vi "RGseriesSerial.vi"() -> ()   [LabVIEW 2009]
uses:
  <vilib>/Instr/_visa.llb/VISA Configure Serial Port (Instr).vi
panel:
  out "ICN MES COM":string
  out "VCN MES COM":string
  in  "On/Off":bool
  out "VCN MES":string
  in  "VISA resource name":refnum<visa-resource-name>
  in  "timeout (10sec)":u32=10000
  out "ICN MES":string
  out "VCN_REQ_COM":string
  out "ICN_REQ_COM":string
  in  "VCN_REQ":dbl
  in  "ICN_REQ":dbl(knob) scale=0.0..3.0
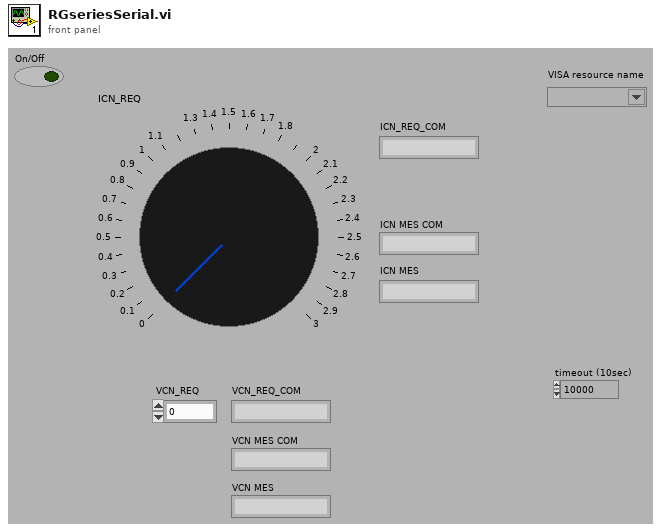
[diagram p1: front panel]
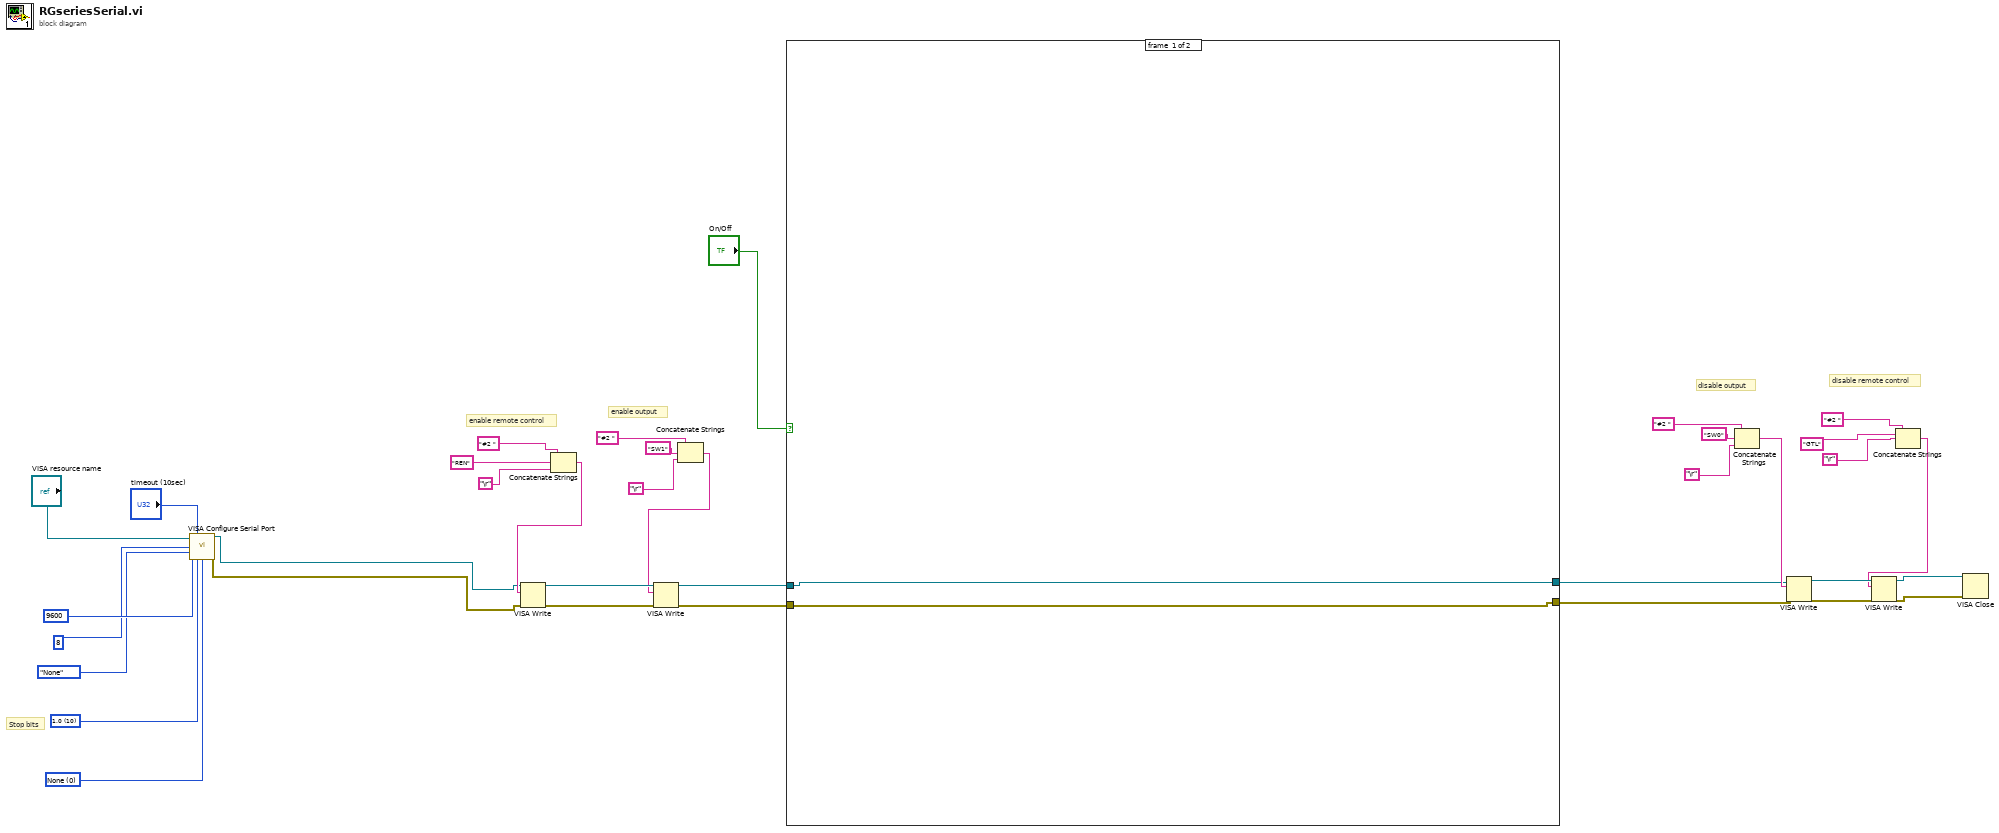
[diagram p0: block diagram]
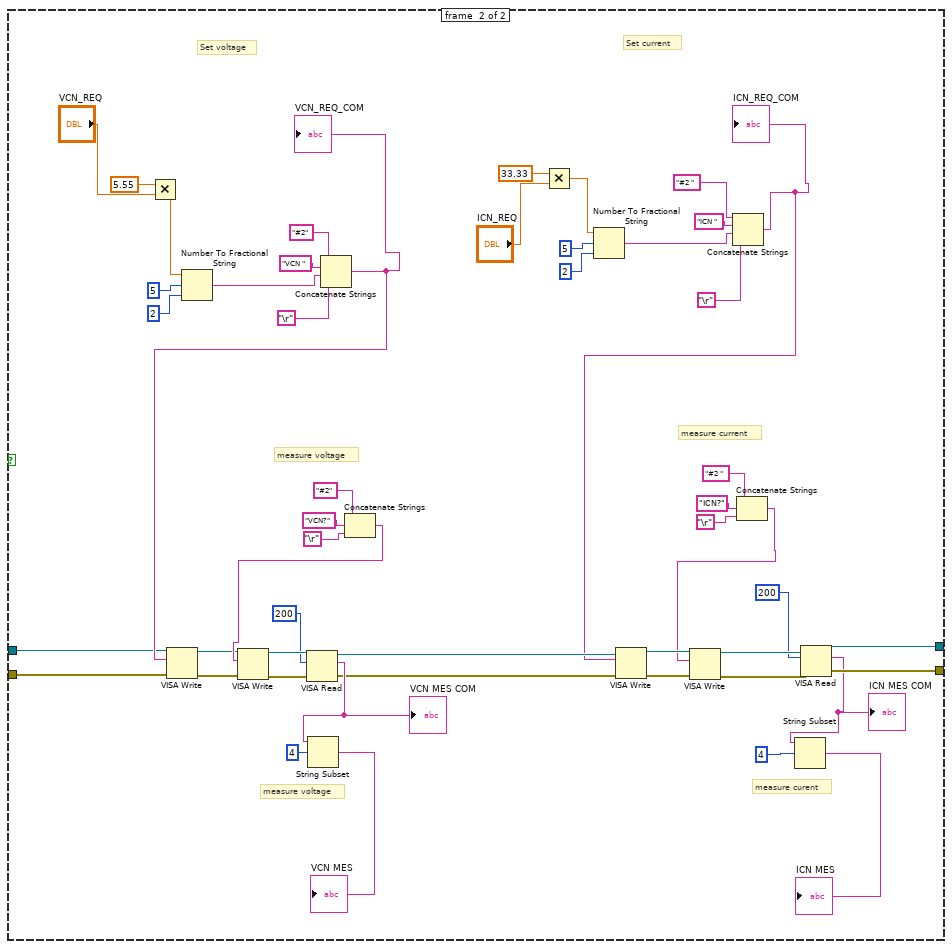
[diagram p2: hidden frame]
diagram:
  w20 = u16 0 items=["None", "XON/XOFF", "RTS/CTS", "XON/XOFF & RTS/CTS", "DTR/DSR", "XON/XOFF & DTR/DSR"] ("flow control (0:none)")
  w21 = u16 10 items=["1.0"=10, "1.5"=15, "2.0"=20] ("stop bits (10: 1 bit)")
  # "Stop bits"
  # "enable remote control"
  # "enable output"
  # "disable remote control"
  # "disable output"
  n1 = call-poly "VISA Configure Serial Port"("VISA resource name"="VISA resource name", "timeout (10sec)"="timeout (10sec)", "baud rate (9600)"=u32 9600, "data bits (8)"=u16 8, "parity (0:none)"=enum16{"None", "Odd", "Even", "Mark", "Space"}."None", "stop bits (10: 1 bit)"=w21, "flow control (0:none)"=w20) -> ("VISA resource name out"=w4:refnum<visa-resource-name>, "error out"=w3:errorcluster)  [unwired: 7 in]
  n2 = Concatenate Strings("#2 " ("initial string"), "REN" ("string"), "\r") -> (w17:string)
  n3 = VISA Write(VISA resource name=w4, write buffer=w17, error in (no error)=w3) -> (VISA resource name out=w19:refnum<visa-resource-name>, error out=w18:errorcluster)  [unwired: 1 out]
  n4 = Concatenate Strings("#2 " ("format string"), "SW1" ("initial string"), "\r" ("input 1")) -> (w16:string)
  n5 = VISA Write(VISA resource name=w19, write buffer=w16, error in (no error)=w18) -> (VISA resource name out=w9:refnum<visa-resource-name>, error out=w8:errorcluster)  [unwired: 1 out]
  n6 = case shown="True" "On/Off" {
    tunnel: w9 -> [w38 w60]
    tunnel: w8 -> [w37 w57]
    tunnel: [w37 w47] -> w7
    tunnel: [w38 w46] -> w6
    frame #0 {
    }
    frame #1 {
      # "measure current"
      # "Set current"
      # "measure voltage"
      # "measure voltage"
      # "Set voltage"
      # "measure curent"
      n7 = Multiply(x=5.55, y="VCN_REQ") -> (x*y=w77:dbl)
      n8 = Number To Fractional String(number=w77, width (-)=i16 5, precision (6)=i16 2) -> (F-format string=w68:string)  [unwired: 1 in]
      n9 = Concatenate Strings("#2" ("format string"), "VCN " ("initial string"), w68, "\r") -> (w66:string)
      "VCN_REQ_COM" <- w66
      n10 = VISA Write(VISA resource name=w60, write buffer=w66, error in (no error)=w57) -> (VISA resource name out=w59:refnum<visa-resource-name>, error out=w56:errorcluster)  [unwired: 1 out]
      n11 = Concatenate Strings("#2" ("format string"), "VCN?" ("initial string"), "\r" ("input 1")) -> (w63:string)
      n12 = VISA Write(VISA resource name=w59, write buffer=w63, error in (no error)=w56) -> (VISA resource name out=w58:refnum<visa-resource-name>, error out=w55:errorcluster)  [unwired: 1 out]
      n13 = VISA Read(VISA resource name=w58, byte count=u32 200, error in (no error)=w55) -> (VISA resource name out=w53:refnum<visa-resource-name>, read buffer=w62:string, error out=w52:errorcluster)  [unwired: 1 out]
      "VCN MES COM" <- w62
      n14 = String Subset(string=w62, offset (0)=4) -> (substring=→"VCN MES":string)  [unwired: 1 in]
      n15 = Multiply(x=33.33, y="ICN_REQ") -> (x*y=w80:dbl)
      n16 = Number To Fractional String(number=w80, width (-)=i16 5, precision (6)=i16 2) -> (F-format string=w70:string)  [unwired: 1 in]
      n17 = Concatenate Strings("#2 " ("initial string"), "ICN " ("initial string"), w70, "\r") -> (w41:string)
      "ICN_REQ_COM" <- w41
      n18 = VISA Write(VISA resource name=w53, write buffer=w41, error in (no error)=w52) -> (VISA resource name out=w50:refnum<visa-resource-name>, error out=w51:errorcluster)  [unwired: 1 out]
      n19 = Concatenate Strings("#2 " ("format string"), "ICN?" ("initial string"), "\r" ("input 1")) -> (w43:string)
      n20 = VISA Write(VISA resource name=w50, write buffer=w43, error in (no error)=w51) -> (VISA resource name out=w49:refnum<visa-resource-name>, error out=w48:errorcluster)  [unwired: 1 out]
      n21 = VISA Read(VISA resource name=w49, byte count=u32 200, error in (no error)=w48) -> (VISA resource name out=w46:refnum<visa-resource-name>, read buffer=w45:string, error out=w47:errorcluster)  [unwired: 1 out]
      "ICN MES COM" <- w45
      n22 = String Subset(string=w45, offset (0)=4) -> (substring=→"ICN MES":string)  [unwired: 1 in]
    }
  }
  n23 = Concatenate Strings("#2 " ("format string"), "SW0" ("initial string"), "\r" ("input 1")) -> (w10:string)
  n24 = VISA Write(VISA resource name=w6, write buffer=w10, error in (no error)=w7) -> (VISA resource name out=w13:refnum<visa-resource-name>, error out=w12:errorcluster)  [unwired: 1 out]
  n25 = Concatenate Strings("#2 " ("initial string"), "\r", "GTL" ("input 1")) -> (w11:string)
  n26 = VISA Write(VISA resource name=w13, write buffer=w11, error in (no error)=w12) -> (VISA resource name out=w14:refnum<visa-resource-name>, error out=w15:errorcluster)  [unwired: 1 out]
  n27 = VISA Close(VISA resource name=w14, error in (no error)=w15) -> ()  [unwired: 1 out]
